vi "MGI SRS Graph Settings.vi"(7 "Command":T1, 8 "Error In":errorcluster, 10 "Graph Info In":T2, 11 "Graph/Chart Ref":refnum<vi>) -> (0 "Error Out":errorcluster, 2 "Graph Info Out":T2)   [LabVIEW 2016]
doc: "Populates the Graph Settings cluster with values from the Graph of the specified Refnum.\n\nAuthored by Shawn Walpole\nsupport@mooregoodideas.com\nwww.mooregoodideas.com\n\nCopyright (c) 2010, Moore Good Ideas, Inc.\n\nAll rights reserved.\n\nRedistribution and use in source and binary forms, with or without modification, are permitted provided that the following conditions are met:\n\n * Redistributions of source code must retain the above copyright notice, this list of conditions and the following disclaimer.\n * Redistributions in binary form must reproduce the above copyright notice, this list of conditions and the following disclaimer in the documentation and/or other materials provided with the distribution.\n * Neither the name of Moore Good Ideas, Inc. nor the names of its contributors may be used to endorse or promote products derived from this software without specific prior written permission.\n\nTHIS SOFTWARE IS PROVIDED BY THE COPYRIGHT HOLDERS AND CONTRIBUTORS \"AS IS\" AND ANY EXPRESS OR IMPLIED WARRANTIES, INCLUDING, BUT NOT LIMITED TO, THE IMPLIED WARRANTIES OF MERCHANTABILITY AND FITNESS FOR A PARTICULAR PURPOSE ARE DISCLAIMED. IN NO EVENT SHALL THE COPYRIGHT OWNER OR CONTRIBUTORS BE LIABLE FOR ANY DIRECT, INDIRECT, INCIDENTAL, SPECIAL, EXEMPLARY, OR CONSEQUENTIAL DAMAGES (INCLUDING, BUT NOT LIMITED TO, PROCUREMENT OF SUBSTITUTE GOODS OR SERVICES; LOSS OF USE, DATA, OR PROFITS; OR BUSINESS INTERRUPTION) HOWEVER CAUSED AND ON ANY THEORY OF LIABILITY, WHETHER IN CONTRACT, STRICT LIABILITY, OR TORT (INCLUDING NEGLIGENCE OR OTHERWISE) ARISING IN ANY WAY OUT OF THE USE OF THIS SOFTWARE, EVEN IF ADVISED OF THE POSSIBILITY OF SUCH DAMAGE."
uses:
  <userlib>/_MGI/Application Control/MGI Save & Restore Settings/MGI SRS Graph Setting Cluster.ctl
  <userlib>/_MGI/Application Control/MGI Save & Restore Settings/MGI SRS Graph Plot Cluster.ctl
  <userlib>/_MGI/Application Control/MGI Save & Restore Settings/MGI SRS Graph Cursor Cluster.ctl
  <userlib>/_MGI/Application Control/MGI Save & Restore Settings/MGI SRS Command Enum.ctl
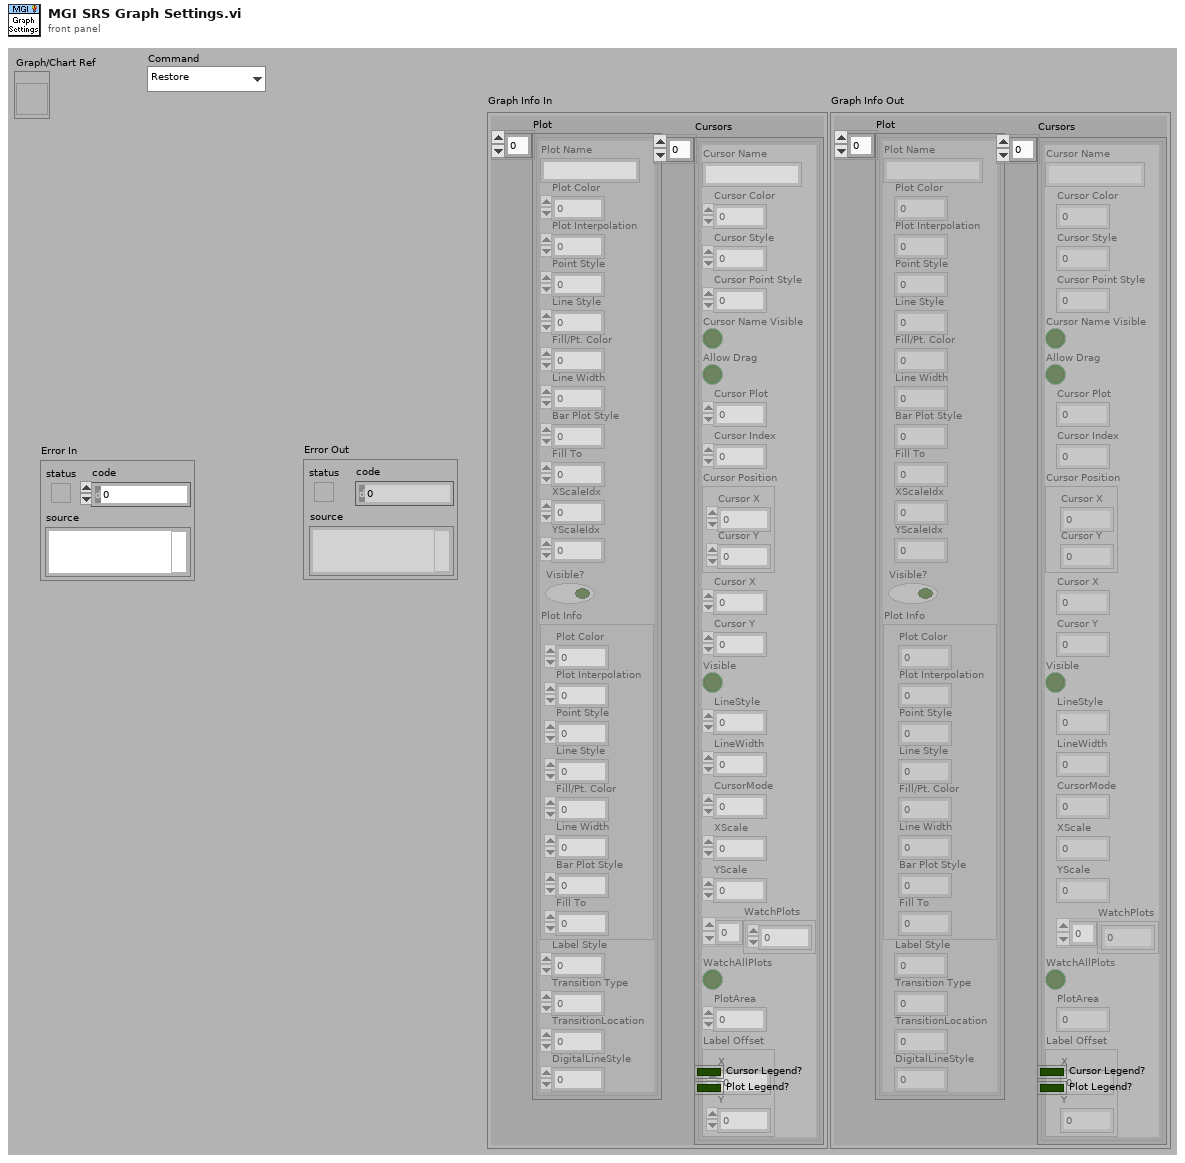
[diagram p1: front panel]
types:
  T1 = typedef "MGI SRS Command Enum.ctl" = enum16{"Restore", "Save"}
  T2 = typedef "MGI SRS Graph Setting Cluster.ctl" = cluster{"Plot":T3[], "Cursors":T4[], "Cursor Legend?":bool, "Plot Legend?":bool}
  T3 = typedef "MGI SRS Graph Plot Cluster.ctl" = cluster{"Plot Name":string, "Plot Color":u32, "Plot Interpolation":u8, "Point Style":u8, "Line Style":u8, "Fill/Pt. Color":u32, "Line Width":u8, "Bar Plot Style":u8, "Fill To":i16, "XScaleIdx":u32, "YScaleIdx":u32, "Visible?":bool, "Plot Info":cluster{"Plot Color":u32, "Plot Interpolation":u8, "Point Style":u8, "Line Style":u8, "Fill/Pt. Color":u32, "Line Width":u8, "Bar Plot Style":u8, "Fill To":i16}, "Label Style":u8, "Transition Type":u8, "TransitionLocation":u8, "DigitalLineStyle":u8}
  T4 = typedef "MGI SRS Graph Cursor Cluster.ctl" = cluster{"Cursor Name":string, "Cursor Color":u32, "Cursor Style":u8, "Cursor Point Style":u8, "Cursor Name Visible":bool, "Allow Drag":bool, "Cursor Plot":i32, "Cursor Index":i32, "Cursor Position":cluster{"Cursor X":dbl, "Cursor Y":dbl}, "Cursor X":dbl, "Cursor Y":dbl, "Visible":bool, "LineStyle":u8, "LineWidth":u8, "CursorMode":u32, "XScale":u32, "YScale":u32, "WatchPlots":i32[], "WatchAllPlots":bool, "PlotArea":i32, "Label Offset":cluster{"X":dbl, "Y":dbl}}
  T5 = cluster{"Name":string, "Color":u32, "Style":u8, "Point Style":u8, "Name Visible":bool, "Allow Drag":bool, "Cursor Mode":u32, "Plot":i32, "Index":i32, "Position":cluster{"X":dbl, "Y":dbl}, "X Scale":u32, "Y Scale":u32, "Watch Plots":i32[], "Watch All Plots":bool, "Plot Area":i32, "Label Offset":cluster{"X":dbl, "Y":dbl}}
  T6 = typedef "LVCursorListTypeDef.ctl" = cluster{"Name":string, "Color":u32, "Style":u8, "Point Style":u8, "Name Visible":bool, "Allow Drag":bool, "Cursor Mode":u32, "Plot":i32, "Index":i32, "Position":cluster{"X":dbl, "Y":dbl}, "X Scale":u32, "Y Scale":u32, "Watch Plots":i32[], "Watch All Plots":bool, "Plot Area":i32, "Label Offset":cluster{"X":dbl, "Y":dbl}}[]
  T7 = typedef "LVPointDoubleTypeDef.ctl" = cluster{"Cursor X":dbl, "Cursor Y":dbl}
  T8 = cluster{"Plot Color":u32, "Plot Interpolation":u8, "Point Style":u8, "Line Style":u8, "Fill/Pt. Color":u32, "Line Width":u8, "Bar Plot Style":u8, "Fill To":i16}
  T9 = cluster{"Visible":bool, "LineStyle":u8, "LineWidth":u8, "CursorMode":u32, "WatchPlots":i32[], "WatchAllPlots":bool, "PlotArea":i32}
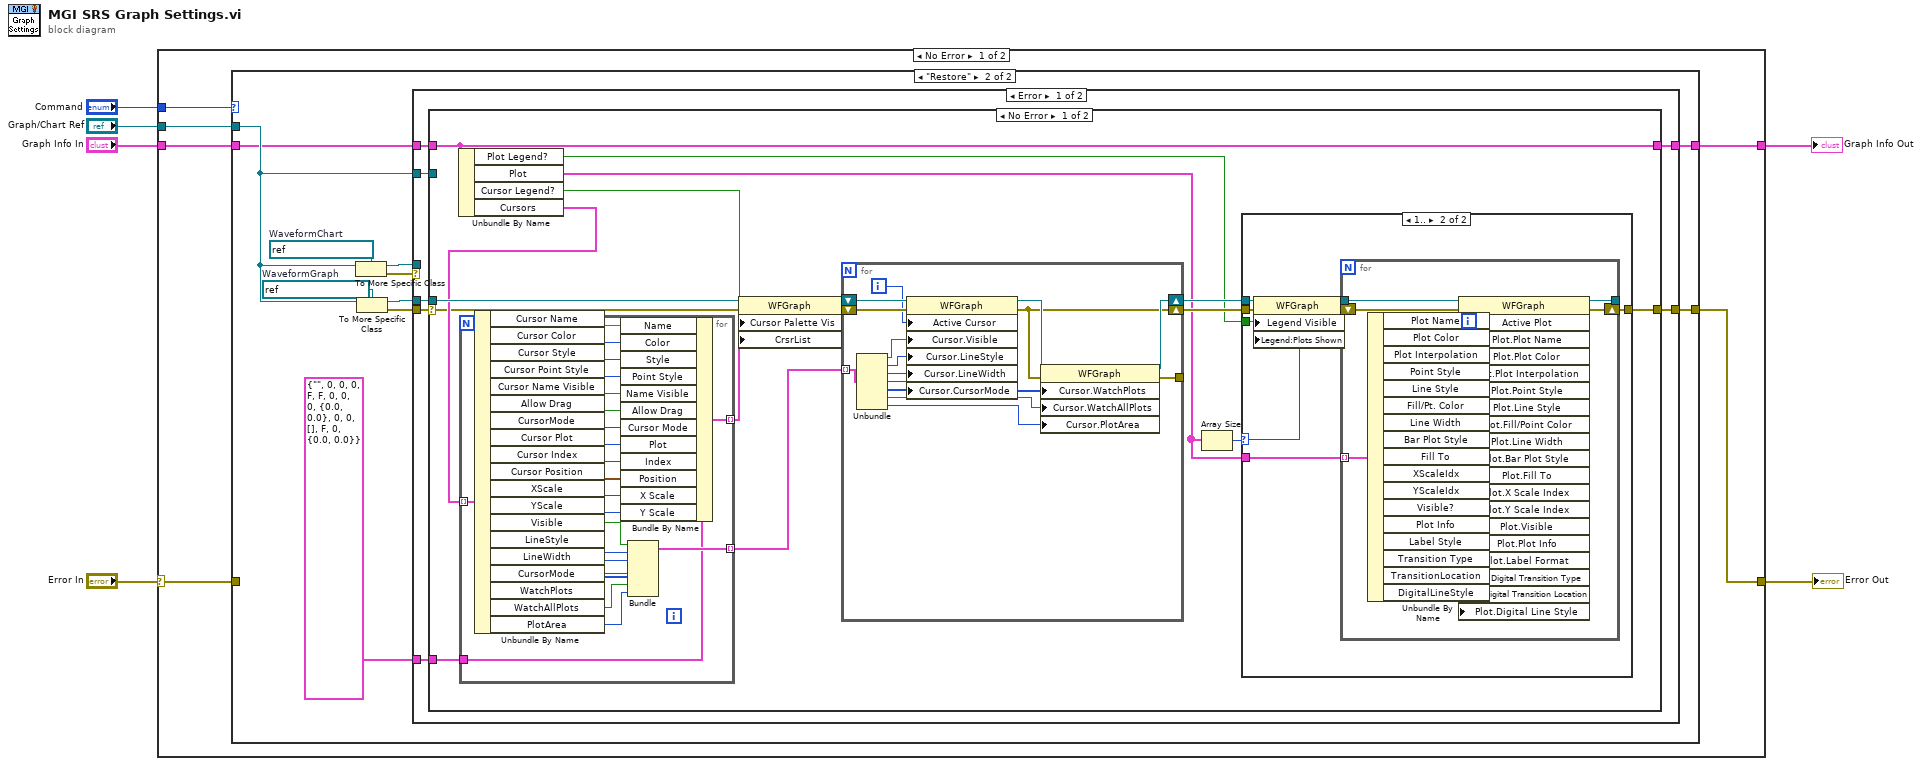
[diagram p0: block diagram]
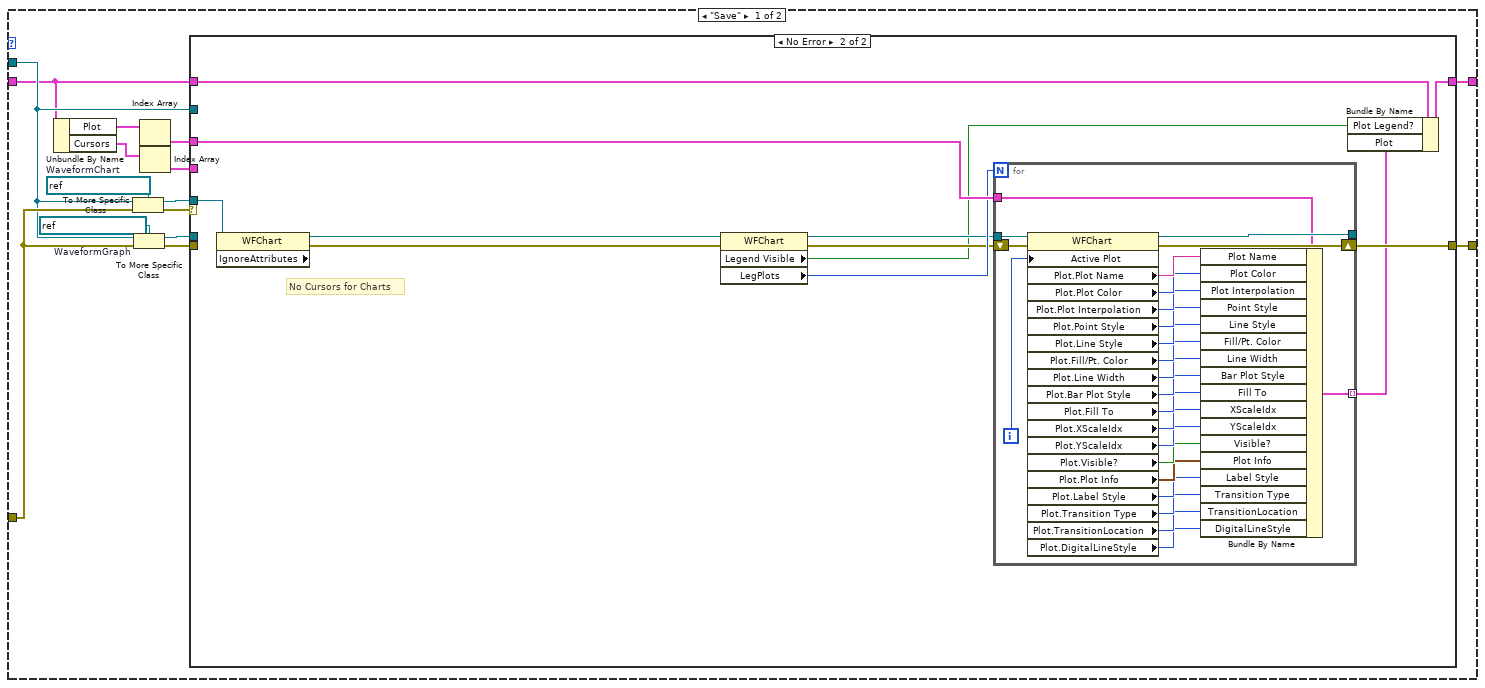
[diagram p2: hidden frame]
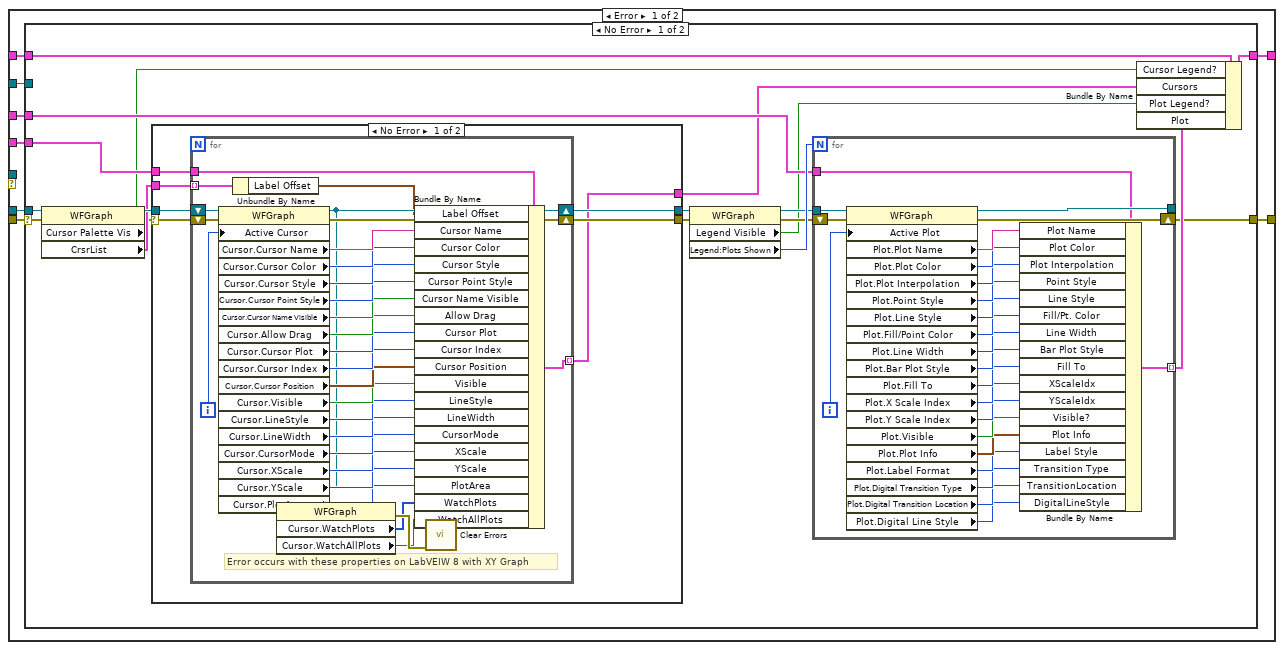
[diagram p3: hidden frame]
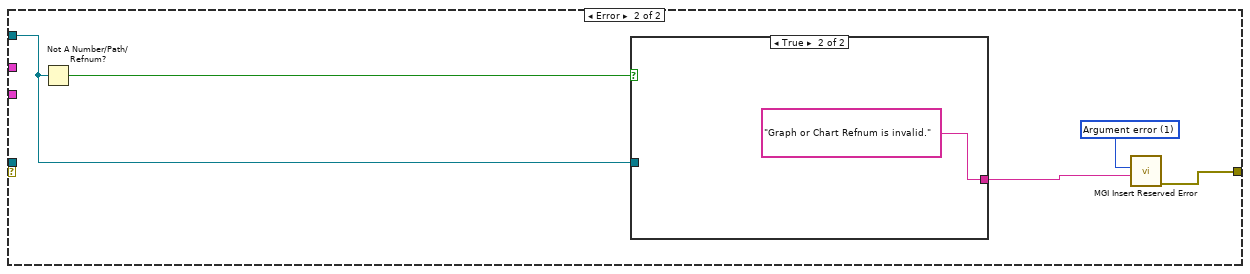
[diagram p5: hidden frame]
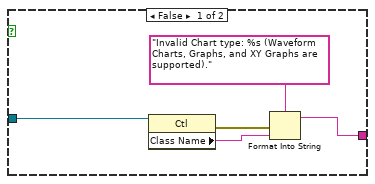
[diagram p6: hidden frame]
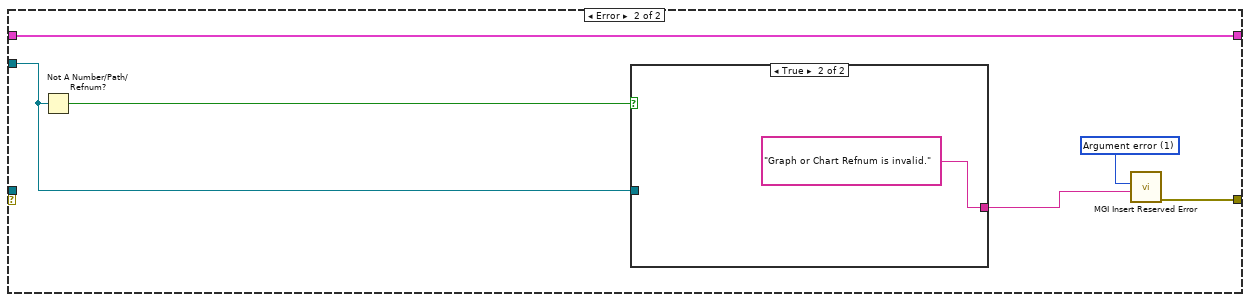
[diagram p8: hidden frame]
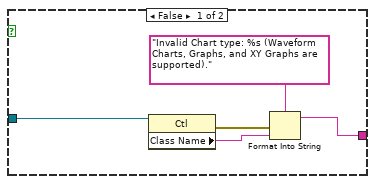
[diagram p9: hidden frame]
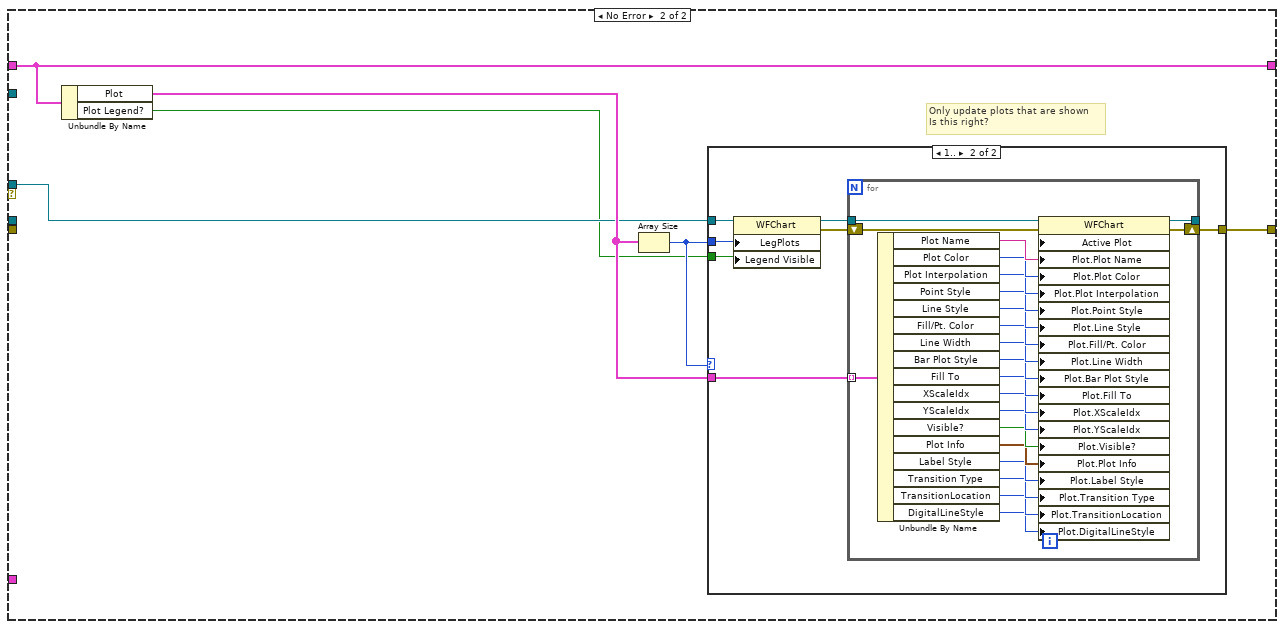
[diagram p10: hidden frame]
diagram:
  n1 = case shown="No Error" "Error In" {
    selector: "Error In" -> [w11 w315]
    tunnel: "Command" -> [w7 _]
    tunnel: "Graph/Chart Ref" -> [w12 _]
    tunnel: "Graph Info In" -> [w10 w314]
    tunnel: [w9 w314] -> w2
    tunnel: [w8 w315] -> w1
    frame No Error {
      n2 = case shown="\"Restore\"" w7 {
        tunnel: w11 -> [w25 _]
        tunnel: w12 -> [w19 w165]
        tunnel: [w21 w167] -> w8
        tunnel: w10 -> [w18 w164]
        tunnel: [w13 w163] -> w9
        frame "Save" {
          w27 = refnum<vi> refnum  # WaveformGraph
          w26 = refnum<vi> refnum  # WaveformChart
          n3 = Unbundle By Name(w18) -> ("Plot"=w17:T3[], "Cursors"=w16:T4[])
          n4 = To More Specific Class(target class=w26, reference=w19, error in=w25) -> (specific class reference=w20:refnum<vi>, error out=w24:errorcluster)
          n5 = To More Specific Class(target class=w27, reference=w19, error in=w25) -> (specific class reference=w22:refnum<vi>, error out=w23:errorcluster)
          n6 = Index Array(array=w17) -> (element=w15:T3)  [unwired: 1 in]
          n7 = Index Array(array=w16) -> (element=w14:T4)  [unwired: 1 in]
          n8 = case shown="No Error" w24 {
            tunnel: w23 -> [w35 _]
            tunnel: w22 -> [w34 _]
            tunnel: [w33 w137] -> w21
            tunnel: w20 -> [_ w129]
            tunnel: w19 -> [w32 _]
            tunnel: w18 -> [w31 w136]
            tunnel: w15 -> [w30 w135]
            tunnel: w14 -> [w29 _]
            tunnel: [w28 w134] -> w13
            frame Error {
              n9 = case shown="No Error" w35 {
                selector: w35 -> [w41 _]
                tunnel: w34 -> [w40 _]
                tunnel: [w48 w118] -> w33
                tunnel: w32 -> [_ w116]
                tunnel: w31 -> [w51 _]
                tunnel: w30 -> [w50 _]
                tunnel: w29 -> [w43 _]
                tunnel: [w47 _] -> w28
                frame No Error {
                  n10 = property class="WFGraph"(reference=w40, error in=w41) -> (reference out=w46:refnum<vi>, error out=w38:errorcluster, "Cursor Palette Vis"=w36:bool, "CrsrList"=w42:T6)
                  n11 = case shown="No Error" w38 {
                    selector: w38 -> [w55 _]
                    tunnel: w46 -> [w61 w90]
                    tunnel: [w60 w90] -> w45
                    tunnel: [w59 _] -> w44
                    tunnel: w43 -> [w58 _]
                    tunnel: w42 -> [w57 _]
                    tunnel: [w56 _] -> w39
                    frame No Error {
                      n12 = for {
                        shift-right: [w87] -> w59
                        shift-left: w55 -> [w89]
                        tunnel: w58 -> [w86]
                        tunnel: [w85] -> w56 mode=indexing
                        shift-right: [w66] -> w60
                        shift-left: w61 -> [w88]
                        tunnel: w57 -> [w63] mode=indexing
                        i -> [w68]
                        # "Error occurs with these properties on LabVEIW 8 with XY Graph"
                        n13 = property class="WFGraph"(reference=w88, error in=w89, "Active Cursor"=w68) -> (reference out=w66:refnum<vi>, error out=w87:errorcluster, "Cursor.Cursor Name"=w84:string, "Cursor.Cursor Color"=w83:u32, "Cursor.Cursor Style"=w82:u8, "Cursor.Cursor Point Style"=w81:u8, "Cursor.Cursor Name Visible"=w80:bool, "Cursor.Allow Drag"=w79:bool, "Cursor.Cursor Plot"=w78:i32, "Cursor.Cursor Index"=w77:i32, "Cursor.Cursor Position"=w76:T7, "Cursor.Visible"=w75:bool, "Cursor.LineStyle"=w74:u8, "Cursor.LineWidth"=w73:u8, "Cursor.CursorMode"=w72:u32, "Cursor.XScale"=w71:u32, "Cursor.YScale"=w70:u32, "Cursor.PlotArea"=w69:i32)
                        n14 = Unbundle By Name(w63) -> ("Label Offset"=w62:cluster{"X":dbl, "Y":dbl})
                        n15 = property class="WFGraph"(reference=w66) -> (error out=w67:errorcluster, "Cursor.WatchPlots"=w65:i32[], "Cursor.WatchAllPlots"=w64:bool)  [unwired: 1 in, 1 out]
                        n16 = Bundle By Name(cluster=w86, "Label Offset"=w62, "Cursor Name"=w84, "Cursor Color"=w83, "Cursor Style"=w82, "Cursor Point Style"=w81, "Cursor Name Visible"=w80, "Allow Drag"=w79, "Cursor Plot"=w78, "Cursor Index"=w77, "Cursor Position"=w76, "Visible"=w75, "LineStyle"=w74, "LineWidth"=w73, "CursorMode"=w72, "XScale"=w71, "YScale"=w70, "PlotArea"=w69, "WatchPlots"=w65, "WatchAllPlots"=w64) -> (w85:T4)
                        n17 = call <vilib>:"Clear Errors.vi"("error in (no error)"=w67) -> ()  [unwired: 5 in, 2 out]
                      }
                    }
                    frame Error {
                    }
                  }
                  n18 = property class="WFGraph"(reference=w45, error in=w44) -> (reference out=w52:refnum<vi>, error out=w53:errorcluster, "Legend Visible"=w37:bool, "Legend:Plots Shown"=w54:u32)
                  n19 = for {
                    N: w54 -> [_]
                    shift-right: [w111] -> w48
                    shift-left: w53 -> [w114]
                    tunnel: w52 -> [w113]
                    tunnel: [w110] -> _
                    tunnel: w50 -> [w109]
                    tunnel: [w91] -> w49 mode=indexing
                    i -> [w112]
                    n20 = property class="WFGraph"(reference=w113, error in=w114, "Active Plot"=w112) -> (reference out=w110:refnum<vi>, error out=w111:errorcluster, "Plot.Plot Name"=w108:string, "Plot.Plot Color"=w107:u32, "Plot.Plot Interpolation"=w106:u8, "Plot.Point Style"=w105:u8, "Plot.Line Style"=w104:u8, "Plot.Fill/Point Color"=w103:u32, "Plot.Line Width"=w102:u8, "Plot.Bar Plot Style"=w101:u8, "Plot.Fill To"=w100:i16, "Plot.X Scale Index"=w99:u32, "Plot.Y Scale Index"=w98:u32, "Plot.Visible"=w97:bool, "Plot.Plot Info"=w96:T8, "Plot.Label Format"=w95:u8, "Plot.Digital Transition Type"=w94:u8, "Plot.Digital Transition Location"=w93:u8, "Plot.Digital Line Style"=w92:u8)
                    n21 = Bundle By Name(cluster=w109, "Plot Name"=w108, "Plot Color"=w107, "Plot Interpolation"=w106, "Point Style"=w105, "Line Style"=w104, "Fill/Pt. Color"=w103, "Line Width"=w102, "Bar Plot Style"=w101, "Fill To"=w100, "XScaleIdx"=w99, "YScaleIdx"=w98, "Visible?"=w97, "Plot Info"=w96, "Label Style"=w95, "Transition Type"=w94, "TransitionLocation"=w93, "DigitalLineStyle"=w92) -> (w91:T3)
                  }
                  n22 = Bundle By Name(cluster=w51, "Cursor Legend?"=w36, "Cursors"=w39, "Plot Legend?"=w37, "Plot"=w49) -> (w47:T2)
                }
                frame Error {
                  w119 = u16 1 items=["No error", "Argument error", "Memory is full", "Out of zone", "End of file", "File already open", "Generic file I/O error", "File not found", "File permission error", "Disk is full", "Duplicate path", "Too many files open", "System feature not enabled", "Resource file not found", "Cannot add resource", "Resource not found", "Image not found", "Image memory error", "Pen does not exist", "Config type invalid", "Config token not found", "Config parse error", "Config memory error", "Bad external code format", "Bad external code offset", "External code not present", "Null window", "Destroy window error", "Null menu", "Print aborted", "Bad print record", "Print driver error", "Windows error during printing", "Memory error during printing", "Print dialog error", "Generic print error", "Invalid device refnum", "Device not found", "Device parameter error", "Device unit error", "Cannot open device", "Device call aborted", "Generic error", "Cancelled by user", "Object ID too low", "Object ID too high", "Object not in heap", "Unknown heap", "Unknown object (invalid DefProc)", "Unknown object (DefProc not in table)", "Message out of range", "Invalid (null) method", "Unknown message", "Manager call not supported", "Bad address", "Network operation in progress", "Network operation timed out", "Connection is busy", "Network attribute not supported", "Network error", "Address in use", "System out of memory", "Connection aborted", "Connection refused", "Not connected", "Already connected", "Connection closed", "Initialization error (interapplication manager)", "Bad occurrence", "Wait on unbound occurrence handler", "Occurrence queue overflow", "Datalog type conflict", "Unused", "Unrecognized type (interapplication manager)", "Memory corrupt", "Failed to make temporary DLL", "Old CIN version", "Drag socket not found", "Failed to load drop-object", "Failed to register OLE object", "Failed to release OLE object", "Format specifier type mismatch", "Unknown format specifier", "Too few format specifiers", "Too many format specifiers", "Scan failed", "Newer CIN version", "OLE Convert", "Runtime menu error", "Password tampered", "Unknown error code"] ("Reserved Error Code")
                  n23 = Not A Number/Path/Refnum?(number/path/refnum=w116) -> (NaN/Path/Refnum?=w115:bool)
                  n24 = case shown="True" w115 {
                    tunnel: [w121 "Graph or Chart Refnum is invalid." ("format string")] -> w117
                    tunnel: w116 -> [w120 _]
                    frame False {
                      n25 = property class="Ctl"(reference=w120) -> (error out=w122:errorcluster, "Class Name"=w124:string)  [unwired: 1 in, 1 out]
                      n26 = Format Into String(format string="Invalid Chart type: %s (Waveform Charts, Graphs, and XY Graphs are supported).", error in=w122, w124) -> (resulting string=w121:string)  [unwired: 1 in, 1 out]
                    }
                    frame True {
                    }
                  }
                  n27 = call <userlib>:"MGI Insert Reserved Error.vi"("Error Description"=w117, "Reserved Error Code (Generic error)"=w119) -> ("Error Out"=w118:errorcluster)  [unwired: 9 in]
                }
              }
            }
            frame No Error {
              # "No Cursors for Charts"
              n28 = property class="WFChart" props=["IgnoreAttributes"](reference=w129) -> (reference out=w127:refnum<vi>, error out=w128:errorcluster)  [unwired: 1 in, 1 out]
              n29 = property class="WFChart"(reference=w127, error in=w128) -> (reference out=w131:refnum<vi>, error out=w132:errorcluster, "Legend Visible"=w126:bool, "LegPlots"=w133:u32)
              n30 = for {
                N: w133 -> [_]
                shift-right: [w158] -> w137
                shift-left: w132 -> [w161]
                tunnel: w131 -> [w160]
                tunnel: [w157] -> _
                tunnel: w135 -> [w156]
                tunnel: [w138] -> w130 mode=indexing
                i -> [w159]
                n31 = property class="WFChart"(reference=w160, error in=w161, "Active Plot"=w159) -> (reference out=w157:refnum<vi>, error out=w158:errorcluster, "Plot.Plot Name"=w155:string, "Plot.Plot Color"=w154:u32, "Plot.Plot Interpolation"=w153:u8, "Plot.Point Style"=w152:u8, "Plot.Line Style"=w151:u8, "Plot.Fill/Pt. Color"=w150:u32, "Plot.Line Width"=w149:u8, "Plot.Bar Plot Style"=w148:u8, "Plot.Fill To"=w147:i16, "Plot.XScaleIdx"=w146:u32, "Plot.YScaleIdx"=w145:u32, "Plot.Visible?"=w144:bool, "Plot.Plot Info"=w143:T8, "Plot.Label Style"=w142:u8, "Plot.Transition Type"=w141:u8, "Plot.TransitionLocation"=w140:u8, "Plot.DigitalLineStyle"=w139:u8)
                n32 = Bundle By Name(cluster=w156, "Plot Name"=w155, "Plot Color"=w154, "Plot Interpolation"=w153, "Point Style"=w152, "Line Style"=w151, "Fill/Pt. Color"=w150, "Line Width"=w149, "Bar Plot Style"=w148, "Fill To"=w147, "XScaleIdx"=w146, "YScaleIdx"=w145, "Visible?"=w144, "Plot Info"=w143, "Label Style"=w142, "Transition Type"=w141, "TransitionLocation"=w140, "DigitalLineStyle"=w139) -> (w138:T3)
              }
              n33 = Bundle By Name(cluster=w136, "Plot Legend?"=w126, "Plot"=w130) -> (w134:T2)
            }
          }
        }
        frame "Restore" {
          w172 = refnum<vi> refnum  # WaveformGraph
          w171 = refnum<vi> refnum  # WaveformChart
          n34 = To More Specific Class(target class=w171, reference=w165) -> (specific class reference=w166:refnum<vi>, error out=w170:errorcluster)  [unwired: 1 in]
          n35 = To More Specific Class(target class=w172, reference=w165) -> (specific class reference=w168:refnum<vi>, error out=w169:errorcluster)  [unwired: 1 in]
          n36 = case shown="Error" w170 {
            tunnel: w169 -> [w179 _]
            tunnel: w168 -> [w178 _]
            tunnel: [w177 w283] -> w167
            tunnel: w166 -> [_ w280]
            tunnel: w165 -> [w176 _]
            tunnel: w164 -> [w175 w282]
            tunnel: [w174 w282] -> w163
            tunnel: T5 {"Name"="", "Color"=0, "Style"=0, "Point Style"=0, "Name Visible"=FALSE, "Allow Drag"=FALSE, "Cursor Mode"=0, "Plot"=0, "Index"=0, "Position"={"X"=0.0, "Y"=0.0}, "X Scale"=0, "Y Scale"=0, "Watch Plots"=[], "Watch All Plots"=FALSE, "Plot Area"=0, "Label Offset"={"X"=0.0, "Y"=0.0}} -> [w173 _]
            frame Error {
              n37 = case shown="No Error" w179 {
                selector: w179 -> [w184 _]
                tunnel: w178 -> [w189 _]
                tunnel: [w195 w270] -> w177
                tunnel: w176 -> [_ w268]
                tunnel: w175 -> [w194 w266]
                tunnel: [w194 w266] -> w174
                tunnel: w173 -> [w193 _]
                frame No Error {
                  n38 = Unbundle By Name(w194) -> ("Plot Legend?"=w180:bool, "Plot"=w183:T3[], "Cursor Legend?"=w181:bool, "Cursors"=w188:T4[])
                  n39 = for {
                    tunnel: w188 -> [w265] mode=indexing
                    tunnel: w193 -> [w259]
                    tunnel: [w260] -> w190 mode=indexing
                    tunnel: [w248] -> w185 mode=indexing
                    n40 = Unbundle By Name(w265) -> ("Cursor Name"=w258:string, "Cursor Color"=w257:u32, "Cursor Style"=w256:u8, "Cursor Point Style"=w255:u8, "Cursor Name Visible"=w254:bool, "Allow Drag"=w253:bool, "CursorMode"=w252:u32, "Cursor Plot"=w251:i32, "Cursor Index"=w250:i32, "Cursor Position"=w249:cluster{"Cursor X":dbl, "Cursor Y":dbl}, "XScale"=w244:u32, "YScale"=w243:u32, "Visible"=w261:bool, "LineStyle"=w262:u8, "LineWidth"=w263:u8, "CursorMode"=w264:u32, "WatchPlots"=w247:i32[], "WatchAllPlots"=w246:bool, "PlotArea"=w245:i32)
                    n41 = Bundle By Name(cluster=w259, "Name"=w258, "Color"=w257, "Style"=w256, "Point Style"=w255, "Name Visible"=w254, "Allow Drag"=w253, "Cursor Mode"=w252, "Plot"=w251, "Index"=w250, "Position"=w249, "X Scale"=w244, "Y Scale"=w243) -> (w248:T5)
                    n42 = Bundle("Visible"=w261, "LineStyle"=w262, "LineWidth"=w263, "CursorMode"=w264, "WatchPlots"=w247, "WatchAllPlots"=w246, "PlotArea"=w245) -> (w260:T9)  [unwired: 1 in]
                  }
                  n43 = property class="WFGraph"(reference=w189, error in=w184, "Cursor Palette Vis"=w181, "CrsrList"=w185) -> (reference out=w187:refnum<vi>, error out=w186:errorcluster)
                  n44 = for {
                    shift-right: [w229] -> w191
                    shift-left: w186 -> [w241]
                    shift-right: [w233] -> w192
                    shift-left: w187 -> [w242]
                    tunnel: w190 -> [w240] mode=indexing
                    tunnel: [w228] -> _
                    i -> [w239]
                    n45 = Unbundle(w240) -> ("Visible"=w235:bool, "LineStyle"=w236:u8, "LineWidth"=w237:u8, "CursorMode"=w238:u32, "WatchPlots"=w232:i32[], "WatchAllPlots"=w231:bool, "PlotArea"=w230:i32)
                    n46 = property class="WFGraph"(reference=w242, error in=w241, "Active Cursor"=w239, "Cursor.Visible"=w235, "Cursor.LineStyle"=w236, "Cursor.LineWidth"=w237, "Cursor.CursorMode"=w238) -> (reference out=w234:refnum<vi>, error out=w229:errorcluster)
                    n47 = property class="WFGraph"(reference=w234, error in=w229, "Cursor.WatchPlots"=w232, "Cursor.WatchAllPlots"=w231, "Cursor.PlotArea"=w230) -> (reference out=w233:refnum<vi>, error out=w228:errorcluster)
                  }
                  n48 = Array Size(array=w183) -> (size(s)=w182:i32)
                  n49 = case shown="1.." w182 {
                    selector: w182 -> [_ w198]
                    tunnel: [w196 w202] -> w195
                    tunnel: w192 -> [_ w201]
                    tunnel: w191 -> [w196 w200]
                    tunnel: w183 -> [_ w199]
                    tunnel: w180 -> [_ w197]
                    frame ..0 {
                      # "If there are no plots, there is likely an error with the file.\nNo op seems safest- setting plot legend to show 0 plots gives error\nShowing/Hiding legend?"
                    }
                    frame 1.. {
                      n50 = property class="WFGraph"(reference=w201, error in=w200, "Legend Visible"=w197, "Legend:Plots Shown"=w198) -> (reference out=w203:refnum<vi>, error out=w204:errorcluster)
                      n51 = for {
                        shift-right: [w224] -> w202
                        shift-left: w204 -> [w227]
                        tunnel: w203 -> [w226]
                        tunnel: [w223] -> _
                        tunnel: w199 -> [w205] mode=indexing
                        i -> [w225]
                        n52 = Unbundle By Name(w205) -> ("Plot Name"=w222:string, "Plot Color"=w221:u32, "Plot Interpolation"=w220:u8, "Point Style"=w219:u8, "Line Style"=w218:u8, "Fill/Pt. Color"=w217:u32, "Line Width"=w216:u8, "Bar Plot Style"=w215:u8, "Fill To"=w214:i16, "XScaleIdx"=w213:u32, "YScaleIdx"=w212:u32, "Visible?"=w211:bool, "Plot Info"=w210:T8, "Label Style"=w209:u8, "Transition Type"=w208:u8, "TransitionLocation"=w207:u8, "DigitalLineStyle"=w206:u8)
                        n53 = property class="WFGraph"(reference=w226, error in=w227, "Active Plot"=w225, "Plot.Plot Name"=w222, "Plot.Plot Color"=w221, "Plot.Plot Interpolation"=w220, "Plot.Point Style"=w219, "Plot.Line Style"=w218, "Plot.Fill/Point Color"=w217, "Plot.Line Width"=w216, "Plot.Bar Plot Style"=w215, "Plot.Fill To"=w214, "Plot.X Scale Index"=w213, "Plot.Y Scale Index"=w212, "Plot.Visible"=w211, "Plot.Plot Info"=w210, "Plot.Label Format"=w209, "Plot.Digital Transition Type"=w208, "Plot.Digital Transition Location"=w207, "Plot.Digital Line Style"=w206) -> (reference out=w223:refnum<vi>, error out=w224:errorcluster)
                      }
                    }
                  }
                }
                frame Error {
                  w271 = u16 1 items=["No error", "Argument error", "Memory is full", "Out of zone", "End of file", "File already open", "Generic file I/O error", "File not found", "File permission error", "Disk is full", "Duplicate path", "Too many files open", "System feature not enabled", "Resource file not found", "Cannot add resource", "Resource not found", "Image not found", "Image memory error", "Pen does not exist", "Config type invalid", "Config token not found", "Config parse error", "Config memory error", "Bad external code format", "Bad external code offset", "External code not present", "Null window", "Destroy window error", "Null menu", "Print aborted", "Bad print record", "Print driver error", "Windows error during printing", "Memory error during printing", "Print dialog error", "Generic print error", "Invalid device refnum", "Device not found", "Device parameter error", "Device unit error", "Cannot open device", "Device call aborted", "Generic error", "Cancelled by user", "Object ID too low", "Object ID too high", "Object not in heap", "Unknown heap", "Unknown object (invalid DefProc)", "Unknown object (DefProc not in table)", "Message out of range", "Invalid (null) method", "Unknown message", "Manager call not supported", "Bad address", "Network operation in progress", "Network operation timed out", "Connection is busy", "Network attribute not supported", "Network error", "Address in use", "System out of memory", "Connection aborted", "Connection refused", "Not connected", "Already connected", "Connection closed", "Initialization error (interapplication manager)", "Bad occurrence", "Wait on unbound occurrence handler", "Occurrence queue overflow", "Datalog type conflict", "Unused", "Unrecognized type (interapplication manager)", "Memory corrupt", "Failed to make temporary DLL", "Old CIN version", "Drag socket not found", "Failed to load drop-object", "Failed to register OLE object", "Failed to release OLE object", "Format specifier type mismatch", "Unknown format specifier", "Too few format specifiers", "Too many format specifiers", "Scan failed", "Newer CIN version", "OLE Convert", "Runtime menu error", "Password tampered", "Unknown error code"] ("Reserved Error Code")
                  n54 = Not A Number/Path/Refnum?(number/path/refnum=w268) -> (NaN/Path/Refnum?=w267:bool)
                  n55 = case shown="True" w267 {
                    tunnel: [w273 "Graph or Chart Refnum is invalid." ("format string")] -> w269
                    tunnel: w268 -> [w272 _]
                    frame False {
                      n56 = property class="Ctl"(reference=w272) -> (error out=w274:errorcluster, "Class Name"=w276:string)  [unwired: 1 in, 1 out]
                      n57 = Format Into String(format string="Invalid Chart type: %s (Waveform Charts, Graphs, and XY Graphs are supported).", error in=w274, w276) -> (resulting string=w273:string)  [unwired: 1 in, 1 out]
                    }
                    frame True {
                    }
                  }
                  n58 = call <userlib>:"MGI Insert Reserved Error.vi"("Error Description"=w269, "Reserved Error Code (Generic error)"=w271) -> ("Error Out"=w270:errorcluster)  [unwired: 9 in]
                }
              }
            }
            frame No Error {
              # "Only update plots that are shown\nIs this right?"
              n59 = Unbundle By Name(w282) -> ("Plot"=w281:T3[], "Plot Legend?"=w278:bool)
              n60 = Array Size(array=w281) -> (size(s)=w279:i32)
              n61 = case shown="1.." w279 {
                tunnel: [_ w290] -> w283
                tunnel: w281 -> [_ w289]
                tunnel: w279 -> [_ w286]
                tunnel: w280 -> [_ w285]
                tunnel: w278 -> [_ w284]
                frame 0, Default {
                }
                frame 1.. {
                  n62 = property class="WFChart"(reference=w285, "LegPlots"=w286, "Legend Visible"=w284) -> (reference out=w287:refnum<vi>, error out=w288:errorcluster)  [unwired: 1 in]
                  n63 = for {
                    shift-right: [w310] -> w290
                    shift-left: w288 -> [w313]
                    tunnel: w287 -> [w312]
                    tunnel: [w309] -> _
                    tunnel: w289 -> [w291] mode=indexing
                    i -> [w311]
                    n64 = Unbundle By Name(w291) -> ("Plot Name"=w308:string, "Plot Color"=w307:u32, "Plot Interpolation"=w306:u8, "Point Style"=w305:u8, "Line Style"=w304:u8, "Fill/Pt. Color"=w303:u32, "Line Width"=w302:u8, "Bar Plot Style"=w301:u8, "Fill To"=w300:i16, "XScaleIdx"=w299:u32, "YScaleIdx"=w298:u32, "Visible?"=w297:bool, "Plot Info"=w296:T8, "Label Style"=w295:u8, "Transition Type"=w294:u8, "TransitionLocation"=w293:u8, "DigitalLineStyle"=w292:u8)
                    n65 = property class="WFChart"(reference=w312, error in=w313, "Active Plot"=w311, "Plot.Plot Name"=w308, "Plot.Plot Color"=w307, "Plot.Plot Interpolation"=w306, "Plot.Point Style"=w305, "Plot.Line Style"=w304, "Plot.Fill/Pt. Color"=w303, "Plot.Line Width"=w302, "Plot.Bar Plot Style"=w301, "Plot.Fill To"=w300, "Plot.XScaleIdx"=w299, "Plot.YScaleIdx"=w298, "Plot.Visible?"=w297, "Plot.Plot Info"=w296, "Plot.Label Style"=w295, "Plot.Transition Type"=w294, "Plot.TransitionLocation"=w293, "Plot.DigitalLineStyle"=w292) -> (reference out=w309:refnum<vi>, error out=w310:errorcluster)
                  }
                }
              }
            }
          }
        }
      }
    }
    frame Error {
    }
  }
  "Graph Info Out" <- w2
  "Error Out" <- w1
